vi "createFile.vi"(8 "error in":errorcluster, 11 "File Path":path) -> (0 "error out":errorcluster, 3 "fileRef":refnum<file>)   [LabVIEW 2024]
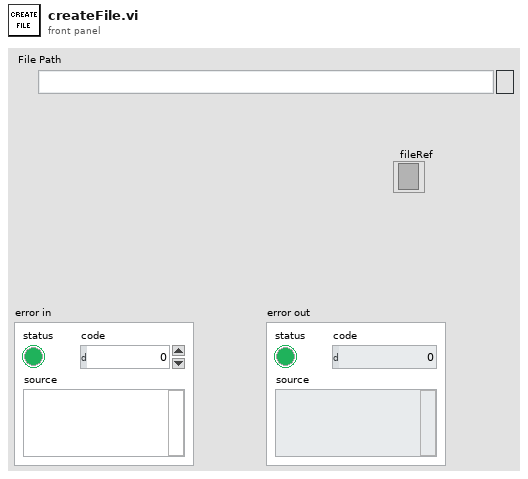
[diagram p1: front panel]
types:
  T1 = enum16{"open", "replace", "create", "open or create", "replace or create", "replace or create with confirmation"}
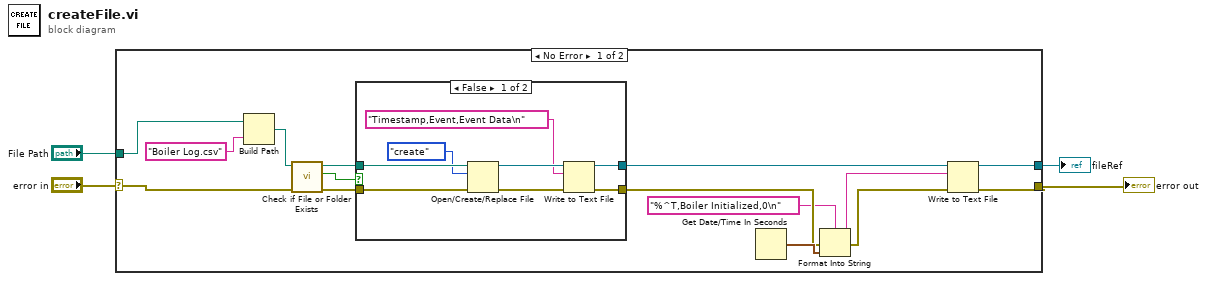
[diagram p0: block diagram]
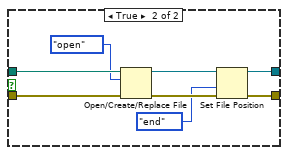
[diagram p2: hidden frame]
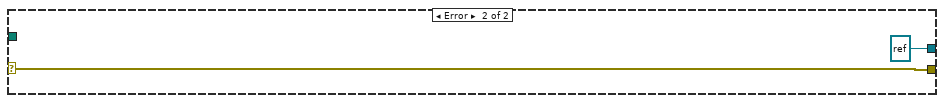
[diagram p3: hidden frame]
diagram:
  n1 = case shown="No Error" "error in" {
    selector: "error in" -> [w17 w37]
    tunnel: [w11 w37] -> w3
    tunnel: "File Path" -> [w19 _]
    tunnel: [w5 refnum<file> refnum ("refnum out")] -> w1
    frame No Error {
      n2 = Build Path(base path=w19, name or relative path="Boiler Log.csv") -> (appended path=w15:path)
      n3 = call <vilib>:"Check if File or Folder Exists.vi"("error in (no error)"=w17, "path"=w15) -> ("error out"=w16:errorcluster, "file or folder exists?"=w14:bool, "dup path"=w13:path)  [unwired: 7 in]
      n4 = case shown="False" w14 {
        tunnel: [w21 w29] -> w12
        tunnel: [w23 w28] -> w9
        tunnel: w16 -> [w27 w34]
        tunnel: w13 -> [w26 w35]
        frame False {
          n5 = Open/Create/Replace File(file path (use dialog)=w26, error in=w27, operation (0:open)=T1."create") -> (refnum out=w22:refnum<file>, error out=w24:errorcluster)  [unwired: 3 in, 1 out]
          n6 = Write to Text File(file (use dialog)=w22, text="Timestamp,Event,Event Data\n", error in=w24) -> (refnum out=w21:refnum<file>, error out=w23:errorcluster)  [unwired: 1 in, 1 out]
        }
        frame True {
          n7 = Open/Create/Replace File(file path (use dialog)=w35, error in=w34, operation (0:open)=T1."open") -> (refnum out=w31:refnum<file>, error out=w32:errorcluster)  [unwired: 3 in, 1 out]
          n8 = Set File Position(refnum=w31, from (0:start)=enum16{"start", "end", "current"}."end", error in=w32) -> (refnum out=w29:refnum<file>, error out=w28:errorcluster)  [unwired: 1 in]
        }
      }
      n9 = Get Date/Time In Seconds() -> (seconds since 1Jan1904=w10:timestamp)
      n10 = Format Into String(format string="%^T,Boiler Initialized,0\n" ("text"), error in=w9, w10) -> (resulting string=w7:string, error out=w8:errorcluster)  [unwired: 1 in]
      n11 = Write to Text File(file (use dialog)=w12, text=w7, error in=w8) -> (refnum out=w5:refnum<file>, error out=w11:errorcluster)  [unwired: 1 in, 1 out]
    }
    frame Error {
    }
  }
  "error out" <- w3
  "fileRef" <- w1
